vi "ConfigureChannel.vi"(2 "channel":u32=8, 3 "input Range (Vpp)":dbl=1.0 format="%.2p", 4 "enable Filter":bool, 5 "ac Coupling":bool) -> (19 "Error Out":errorcluster)   [LabVIEW 2015]
doc: "Configures device parameters for an NI 5170/5171"
uses:
  OscopeAPI/Device Session.lvclass
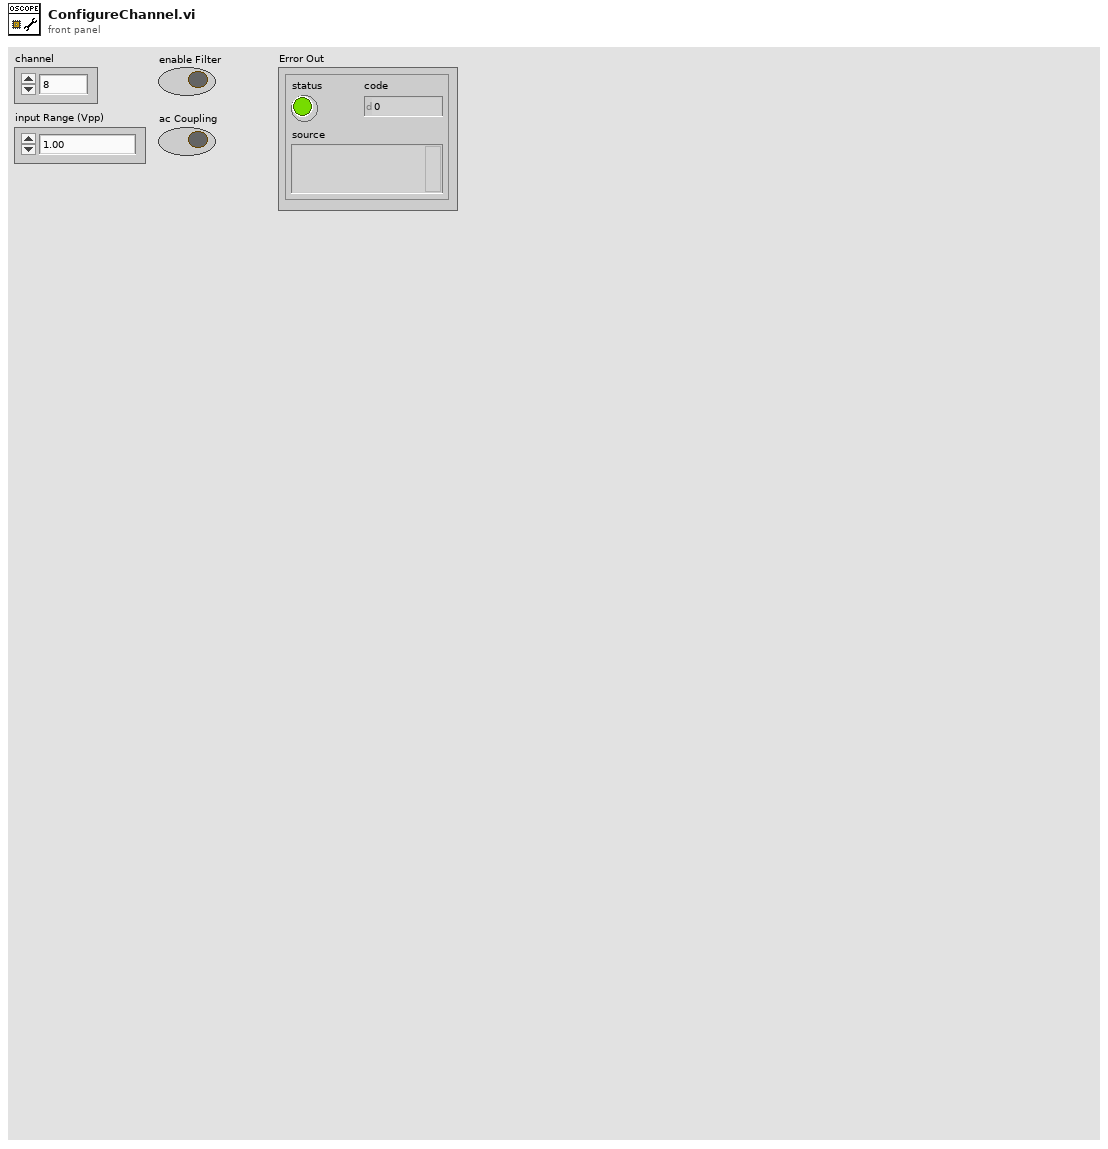
[diagram p1: front panel]
types:
  T1 = enum8{"Default", "Full Bandwidth", "Anti-alias Filter"}
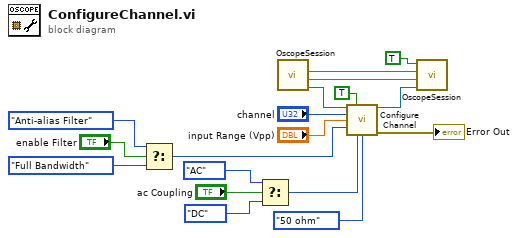
[diagram p0: block diagram]
diagram:
  n1 = Select(t=T1."Anti-alias Filter" ("Bandwidth"), s="enable Filter", f=T1."Full Bandwidth" ("Bandwidth")) -> (s? t:f=w11:T1)
  n2 = Select(t=enum8{"Default", "DC", "AC"}."AC" ("coupling"), s="ac Coupling", f=enum8{"Default", "DC", "AC"}."DC") -> (s? t:f=w8:enum8{"Default", "DC", "AC"})
  n3 = call "OscopeSession.vi"() -> ("Session Out"=w4:refnum<class "Device Session.lvclass">, "Bitfile Path Out"=w5:string, "Device Address Out"=w6:string)  [unwired: 9 in]
  n4 = call "Configure Channel.vi"("device session in"=w4, "enable channel (T)"=TRUE ("enable channel"), "channel"="channel", "vertical range (Vpp)"="input Range (Vpp)", "bandwidth"=w11, "coupling"=w8, "impedance"=enum8{"Default", "1 mega ohm", "50 ohm"}."50 ohm") -> ("device session out"=w17:refnum<class "Device Session.lvclass">, "error out"=→"Error Out":errorcluster)  [unwired: 6 in, 1 out]
  n5 = call "OscopeSession.vi"("Session In"=w17, "Bitfile Path In"=w5, "Device Address In"=w6, "Write"=TRUE) -> ()  [unwired: 5 in, 3 out]
